vi "User Console - Init.vi"(8 "error in (no error)":errorcluster, 11 "User Console":T1) -> (0 "error out":errorcluster, 3 "User Console":T1)   [LabVIEW 2017]
doc: "Initialize all GUI controls of User Console using their referencies."
uses:
  Controls/User Console.ctl
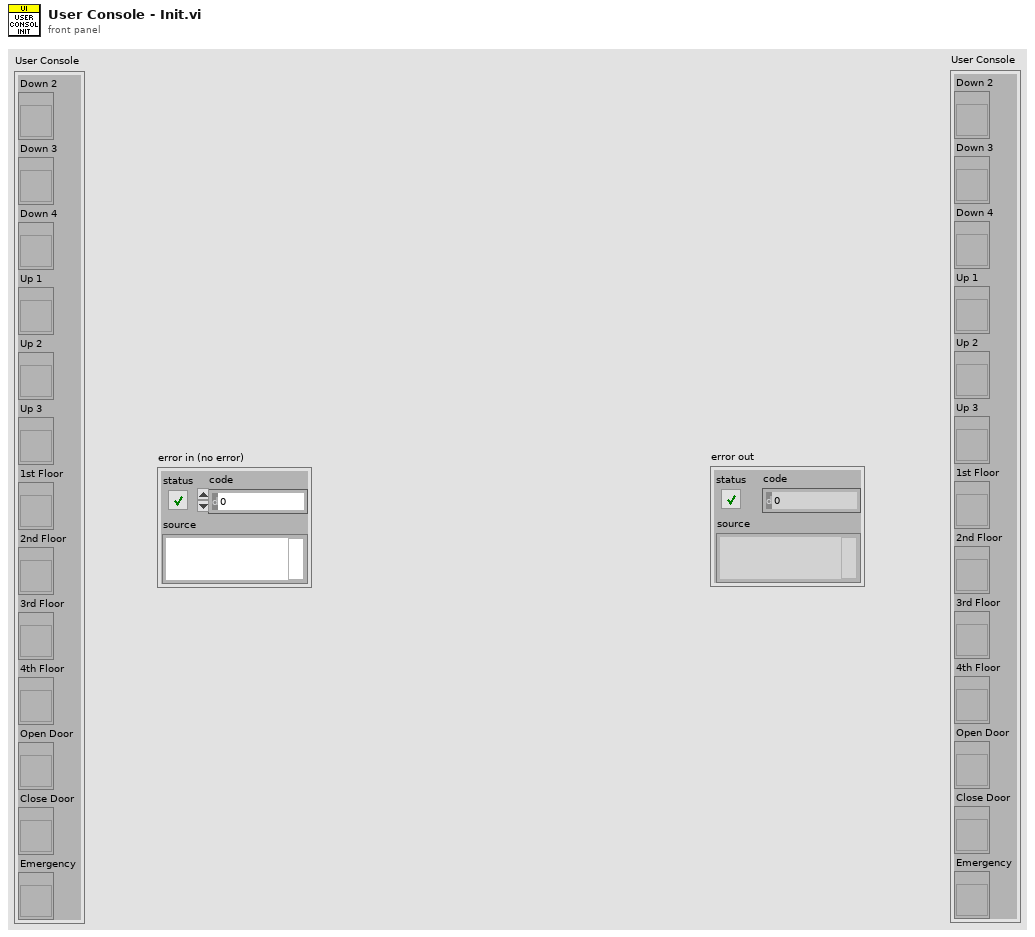
[diagram p1: front panel]
types:
  T1 = typedef "User Console.ctl" = cluster{"Down 2":refnum<vi>, "Down 3":refnum<vi>, "Down 4":refnum<vi>, "Up 1":refnum<vi>, "Up 2":refnum<vi>, "Up 3":refnum<vi>, "1st Floor":refnum<vi>, "2nd Floor":refnum<vi>, "3rd Floor":refnum<vi>, "4th Floor":refnum<vi>, "Open Door":refnum<vi>, "Close Door":refnum<vi>, "Emergency":refnum<vi>}
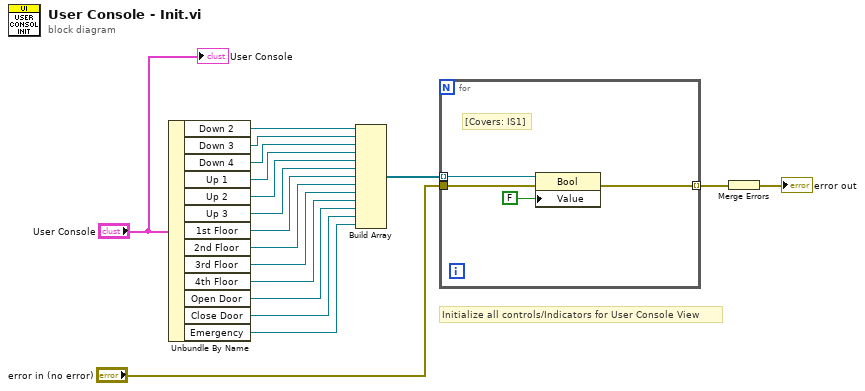
[diagram p0: block diagram]
diagram:
  # "Initialize all controls/Indicators for User Console View"
  n1 = Unbundle By Name("User Console") -> ("Down 2"=w18:refnum<vi>, "Down 3"=w17:refnum<vi>, "Down 4"=w16:refnum<vi>, "Up 1"=w15:refnum<vi>, "Up 2"=w14:refnum<vi>, "Up 3"=w13:refnum<vi>, "1st Floor"=w12:refnum<vi>, "2nd Floor"=w11:refnum<vi>, "3rd Floor"=w10:refnum<vi>, "4th Floor"=w9:refnum<vi>, "Open Door"=w8:refnum<vi>, "Close Door"=w7:refnum<vi>, "Emergency"=w6:refnum<vi>)
  n2 = Build Array(w18, w17, w16, w15, w14, w13, w12, w11, w10, w9, w8, w7, w6) -> (w5:refnum<vi>[])
  n3 = for {
    tunnel: w5 -> [w22] mode=indexing
    tunnel: "error in (no error)" -> [w21]
    tunnel: [w19] -> w4 mode=indexing
    # "[Covers: IS1]"
    n4 = property class="Bool"(reference=w22, error in=w21, "Value"=FALSE) -> (error out=w19:errorcluster)  [unwired: 1 out]
  }
  n5 = Merge Errors(w4) -> (→"error out":errorcluster)
  "User Console" <- "User Console"
